vi "PictureParamsPre.vi"(1 "error out 2":errorcluster, 2 "Picture_Parameter":enum16{"Maximized", "Averaged", "Normalized"}(ring)) -> (0 "error out":errorcluster)   [LabVIEW 2011]
panel:
  in  "Picture_Parameter_Out 3":T1
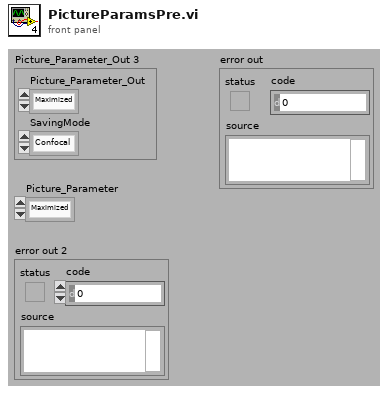
[diagram p1: front panel]
types:
  T1 = cluster{"Picture_Parameter_Out":enum16{"Maximized", "Averaged", "Normalized"}, "SavingMode":enum32{"Confocal", "HighRes", "Video", "Picture", "IntensityTrace", "Test"}}
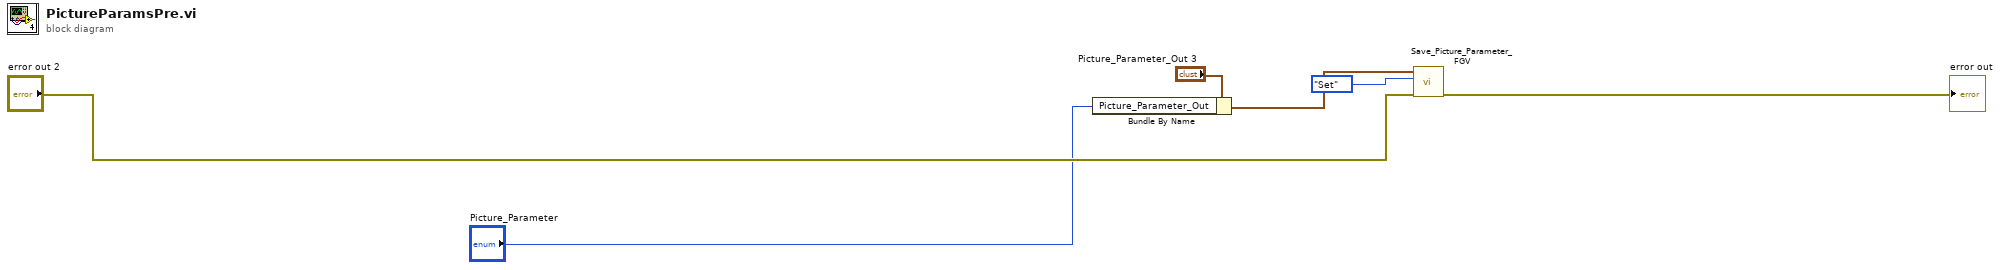
[diagram p0: block diagram]
diagram:
  n1 = Bundle By Name(cluster="Picture_Parameter_Out 3", "Picture_Parameter_Out"="Picture_Parameter") -> (w2:T1)
  n2 = call "Save_Picture_Parameter_FGV.vi"("error in"="error out 2", "FGV_Control"=enum16{"Set", "Get"}."Set", "Picture_Parameter_In"=w2) -> ("error out"=→"error out":errorcluster)  [unwired: 7 in, 1 out]
